vi "题目2.vi"() -> ()   [LabVIEW 2017]
uses:
  <vilib>/Waveform/WDTFileIO.llb/ Write Waveform to File.vi
  <vilib>/Waveform/WDTFileIO.llb/Read Waveform from File.vi
  <vilib>/measure/NI_MABase.lvlib
panel:
  out "波形图":waveform(dbl)[](graph)
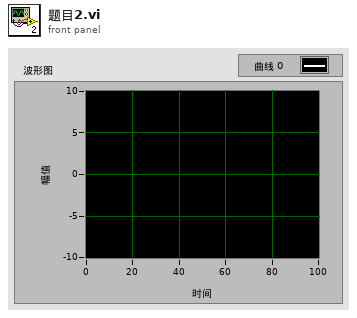
[diagram p1: front panel]
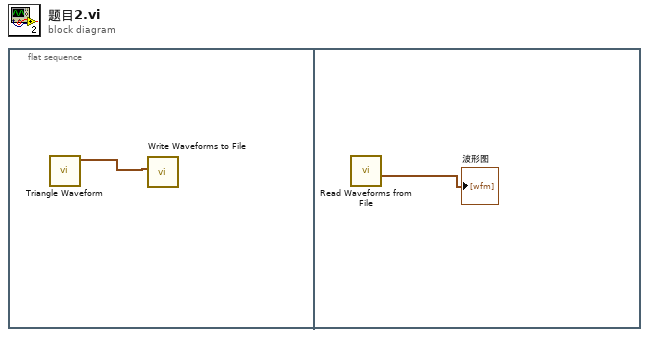
[diagram p0: block diagram]
diagram:
  n1 = flat-sequence {
    frame #0 {
      n2 = call <vilib>:"Triangle Waveform.vi"() -> ("signal out"=w1:waveform(dbl))  [unwired: 10 in, 1 out]
      n3 = call-poly <vilib>:"Write Waveforms to File.vi"("waveform"=w1) -> ()  [unwired: 9 in, 2 out]
    }
    frame #1 {
      n4 = call-poly <vilib>:"Read Waveforms from File.vi"() -> ("all waveforms in record"=→"波形图":waveform(dbl)[])  [unwired: 6 in, 3 out]
    }
  }
